vi "config_file_path.vi"(8 "error in":errorcluster, 10 "reference cluster in":T1) -> (0 "error out":errorcluster, 2 "reference cluster out":T1, 3 "path":path)   [LabVIEW 2016]
uses:
  Type Definitions/reference_cluster.ctl
  Type Definitions/vars_settings.ctl
  Type Definitions/stim_type.ctl
  Type Definitions/vars_runtime.ctl
  Type Definitions/data.ctl
  Type Definitions/notifier_elements_GUI.ctl
  Type Definitions/notifier_elements_DAQ.ctl
  Type Definitions/notifier_elements_write.ctl
  Type Definitions/control_references.ctl
  <vilib>/Utility/sysdir.llb/System Directory Type.ctl
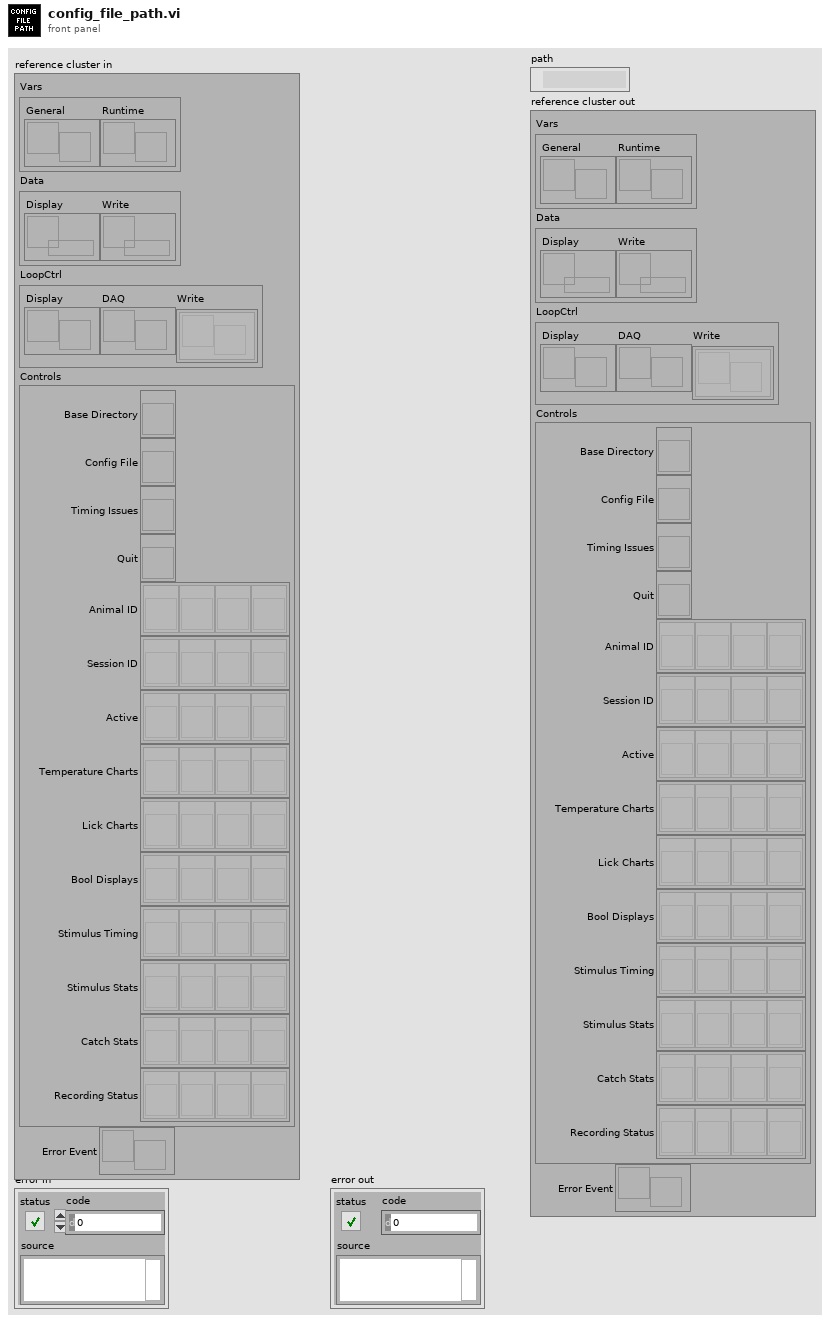
[diagram p1: front panel]
types:
  T1 = typedef "reference_cluster.ctl" = cluster{"Vars":cluster{"General":refnum<notifier>, "Runtime":refnum<notifier>}, "Data":cluster{"Display":refnum<queue>, "Write":refnum<queue>}, "LoopCtrl":cluster{"Display":refnum<notifier>, "DAQ":refnum<notifier>, "Write":refnum<notifier>[]}, "Controls":T2, "Error Event":refnum<user-event>}
  T2 = typedef "control_references.ctl" = cluster{"Base Directory":refnum<vi>, "Config File":refnum<vi>, "Timing Issues":refnum<vi>, "Quit":refnum<vi>, "Animal ID":refnum<vi>[], "Session ID":refnum<vi>[], "Active":refnum<vi>[], "Temperature Charts":refnum<vi>[], "Lick Charts":refnum<vi>[], "Bool Displays":refnum<vi>[], "Stimulus Timing":refnum<vi>[], "Stimulus Stats":refnum<vi>[], "Catch Stats":refnum<vi>[], "Recording Status":refnum<vi>[]}
  T3 = typedef "System Directory Type.ctl" = i32
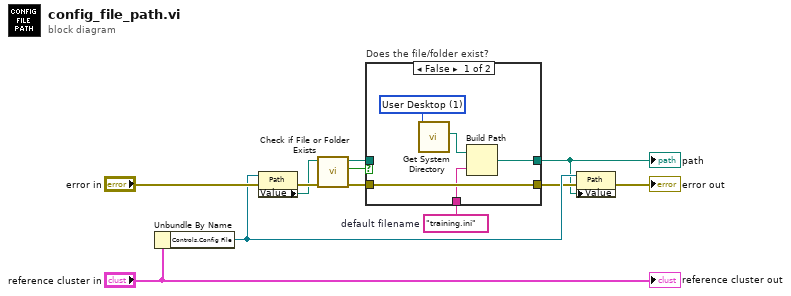
[diagram p0: block diagram]
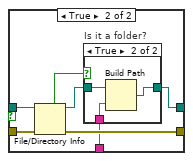
[diagram p2: hidden frame]
diagram:
  w10 = "training.ini"  # default filename
  n1 = Unbundle By Name("reference cluster in") -> ("Controls.Config File"=w4:refnum<vi>)
  n2 = property class="Path"(reference=w4, error in="error in") -> (error out=w11:errorcluster, "Value"=w6:path)  [unwired: 1 out]
  n3 = call <vilib>:"Check if File or Folder Exists.vi"("error in (no error)"=w11, "path"=w6) -> ("error out"=w8:errorcluster, "file or folder exists?"=w9:bool, "dup path"=w7:path)  [unwired: 7 in]
  n4 = case "Does the file/folder exist?" shown="False" w9 {
    tunnel: w7 -> [_ w22]
    tunnel: w8 -> [w17 w21]
    tunnel: [w17 w20] -> w3
    tunnel: [w13 w19] -> w1
    tunnel: w10 -> [w14 w18]
    frame False {
      w15 = T3 1 items=["User Home"=0, "User Desktop"=1, "User Documents"=2, "User Application Data"=3, "User Preferences"=4, "User Temporary"=5, "Public Documents"=6, "Public Application Data"=7, "Public Preferences"=8, "Public Cache"=13, "System Core Libraries"=9, "System Installed Libraries"=10, "Application Files"=11, "Boot Volume Root"=12] ("system directory type")
      # "Use default"
      n5 = call <vilib>:"Get System Directory.vi"("system directory type"=w15) -> ("system directory"=w16:path)  [unwired: 10 in]
      n6 = Build Path(base path=w16, name or relative path=w14) -> (appended path=w13:path)
    }
    frame True {
      n7 = File/Directory Info(path=w22, error in=w21) -> (path out=w23:path, directory=w24:bool, error out=w20:errorcluster)  [unwired: 4 out]
      n8 = case "Is it a folder?" shown="True" w24 {
        tunnel: w23 -> [w25 w28]
        tunnel: w18 -> [_ w27]
        tunnel: [w25 w26] -> w19
        frame False {
        }
        frame True {
          n9 = Build Path(base path=w28, name or relative path=w27) -> (appended path=w26:path)
        }
      }
    }
  }
  "path" <- w1
  n10 = property class="Path"(reference=w4, error in=w3, "Value"=w1) -> (error out=→"error out":errorcluster)  [unwired: 1 out]
  "reference cluster out" <- "reference cluster in"
